vi "test6.4-RegisterInterruptAsStatusFromNonCSM.vi"(8 "error in (no error)":errorcluster, 11 "TestCase in":refnum<class "testcase-CSMBroadcast.lvclass">) -> (0 "error out":errorcluster, 3 "TestCase out":refnum<class "testcase-CSMBroadcast.lvclass">)   [LabVIEW 2017, in "testcase-CSMBroadcast.lvclass"]
uses:
  testcase-CSMBroadcast.lvclass
  src/user.lib/_NEVSTOP/Communicable State Machine(CSM)/AdvanceAPI/CSM - Broadcast Message Type.ctl
  <vilib>/addons/_JKI Toolkits/VI Tester/TestCase.llb/TestCase.lvclass
  src/user.lib/_NEVSTOP/Communicable State Machine(CSM)/Communicable State Machine.lvlib
  CSM/CSM-Testcase.lvlib
  C:/Program Files (x86)/National Instruments/LabVIEW 2017/vi.lib/addons/_JKI Toolkits/VI Tester/TestCase.llb/TestCase.lvclass
panel:
  out "output cluster":T1
  out "LoopCount":i32
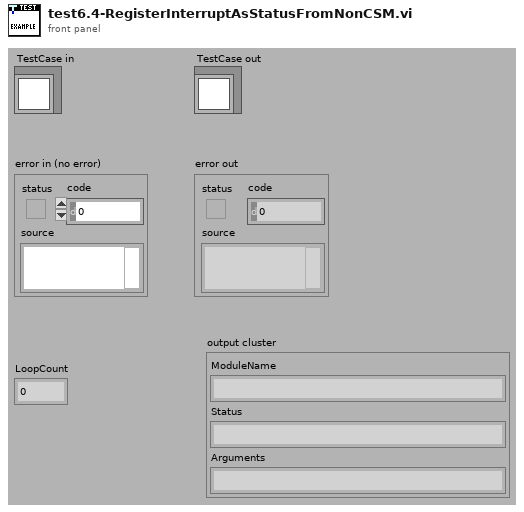
[diagram p1: front panel]
types:
  T1 = cluster{"ModuleName":string, "Status":string, "Arguments":string}
  T2 = typedef "Communicable State Machine.lvlib/CSM - Broadcast Message Type.ctl" = enum16{"<Null>", "Status", "Interrupt"}
  T3 = cluster{"Status Event":refnum<user-event>, "Interrupt Event":refnum<user-event>}
  T4 = cluster{"cluster":cluster{"ModuleName":string, "Status":string, "Arguments":string}}
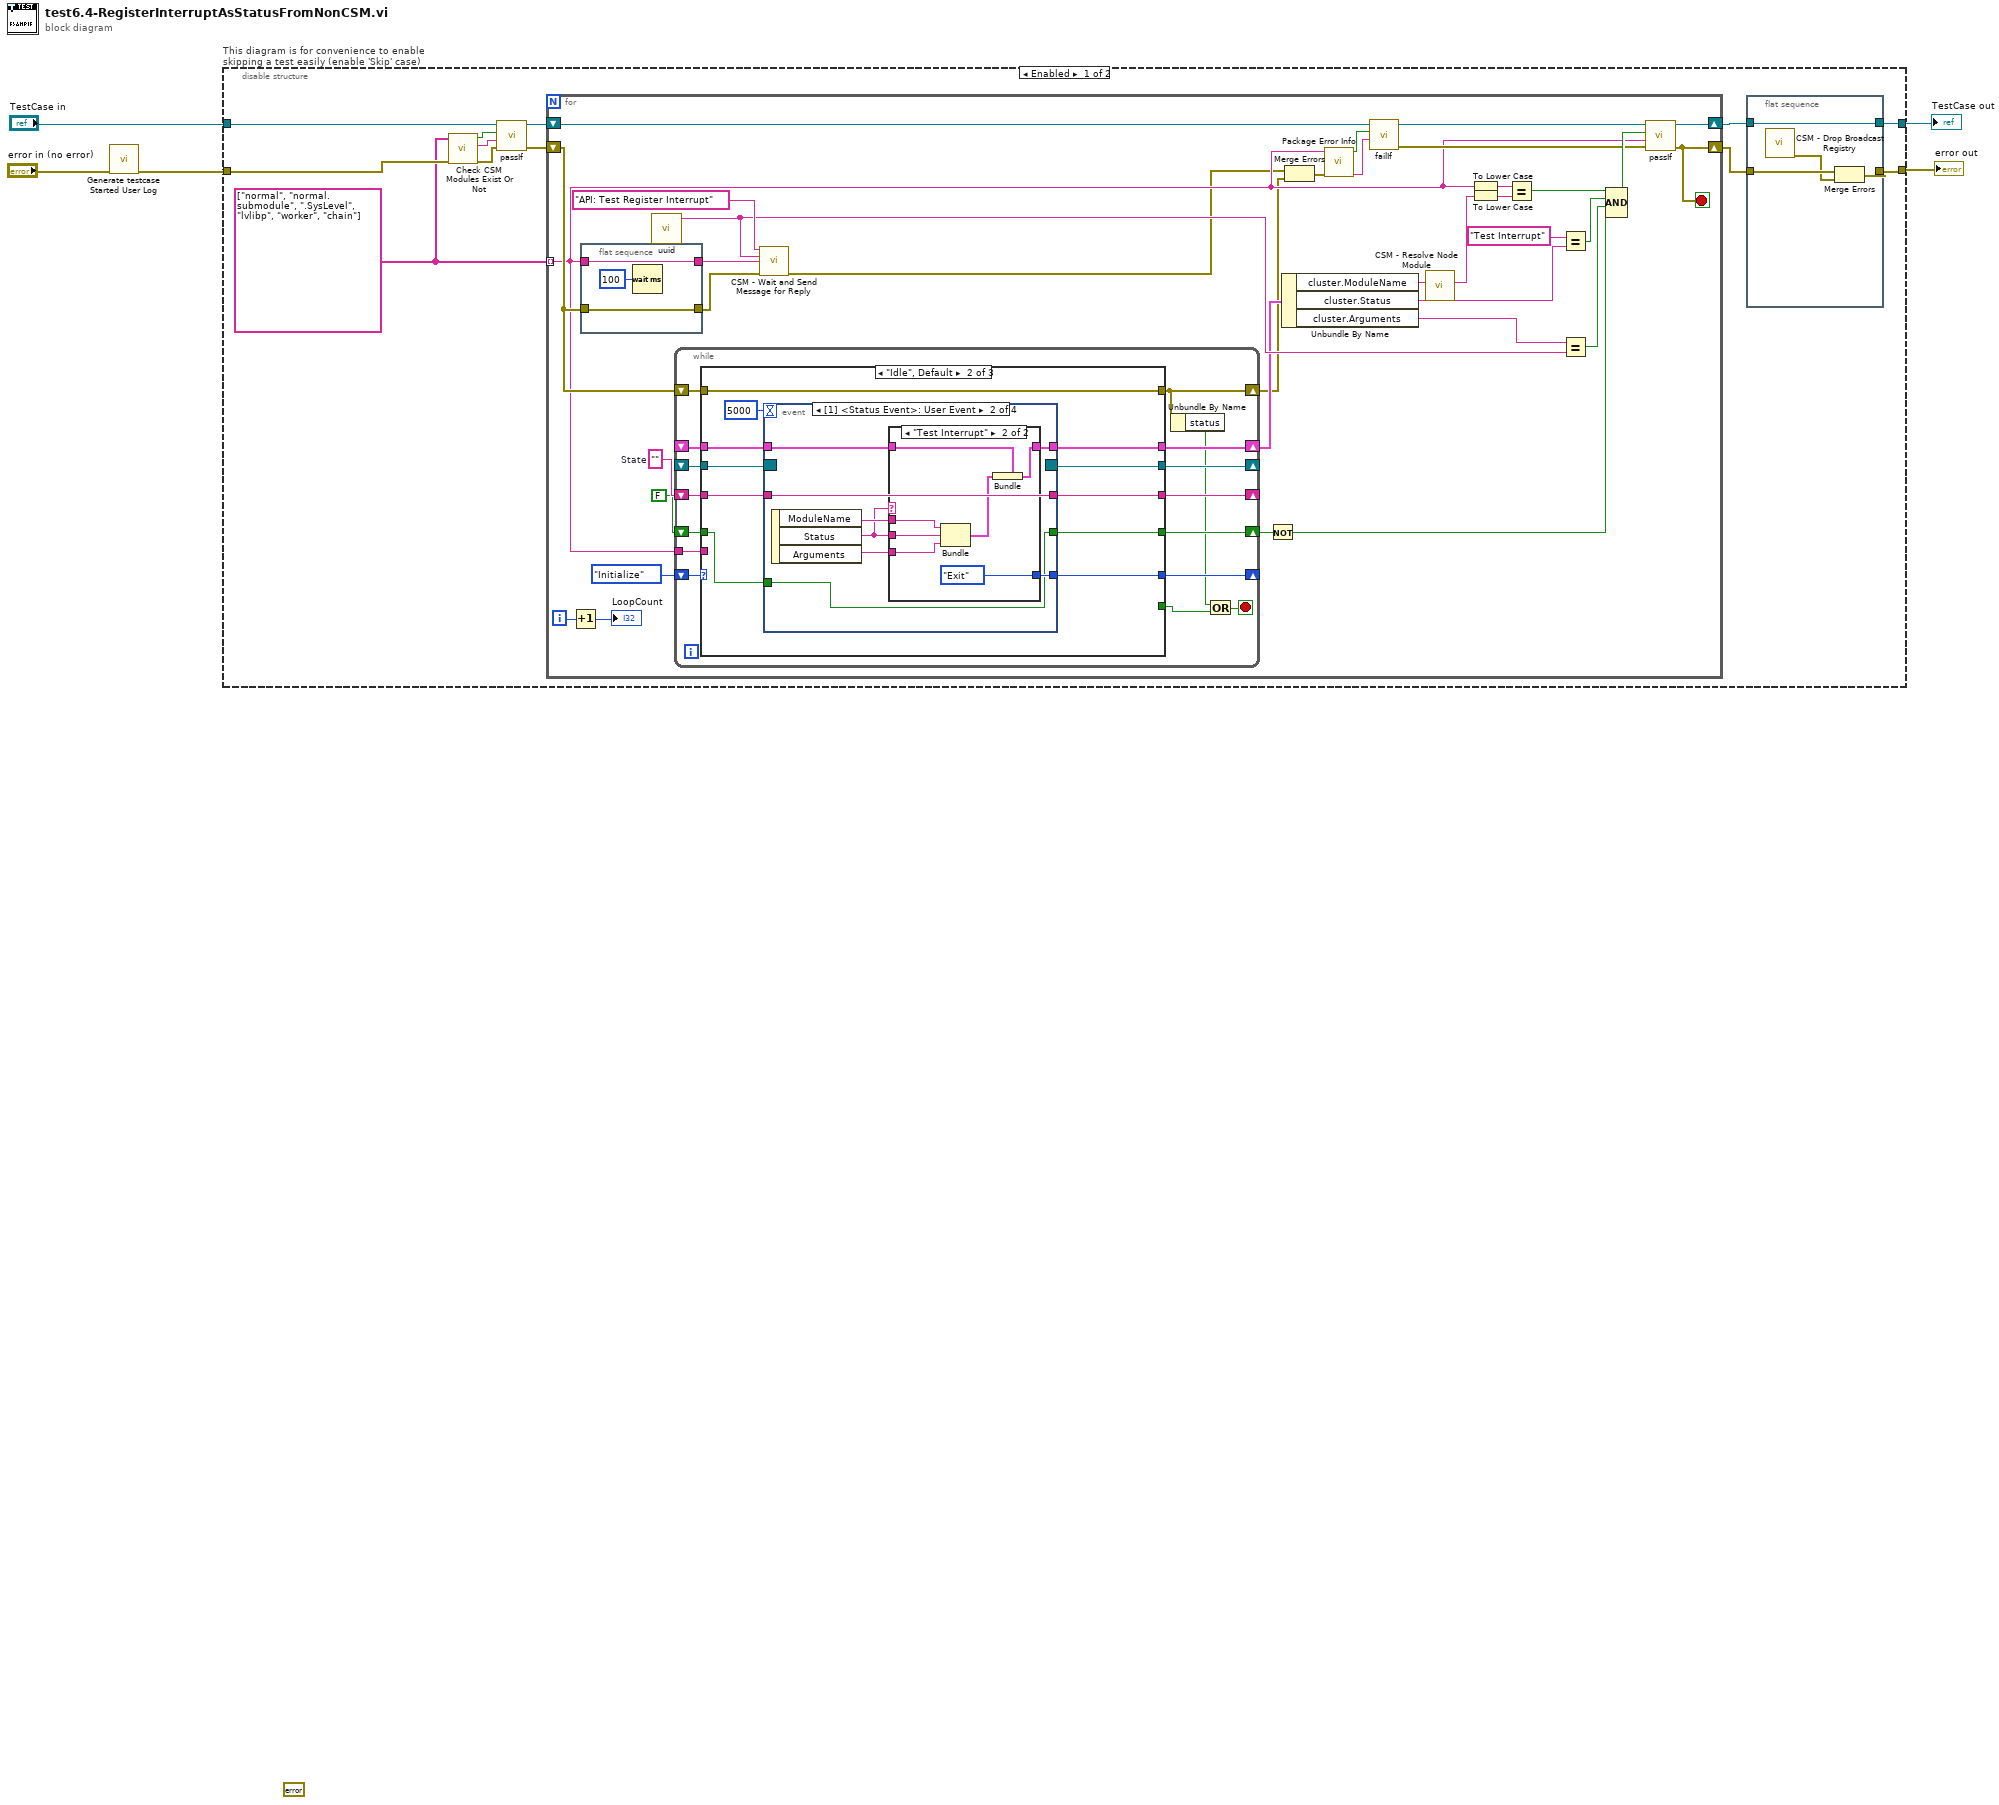
[diagram p0: block diagram]
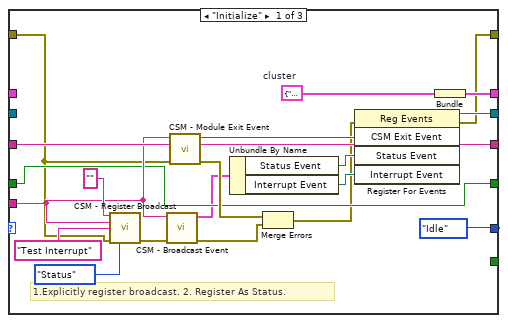
[diagram p2: hidden frame]
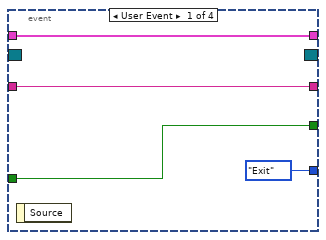
[diagram p3: hidden frame]
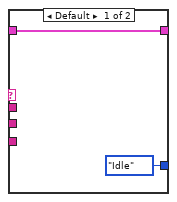
[diagram p4: hidden frame]
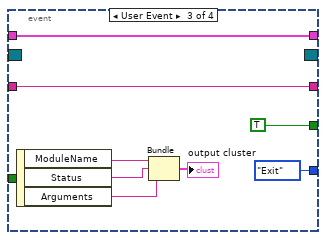
[diagram p5: hidden frame]
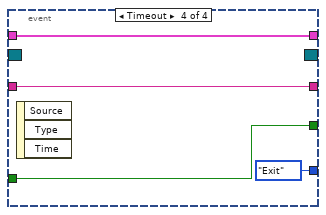
[diagram p6: hidden frame]
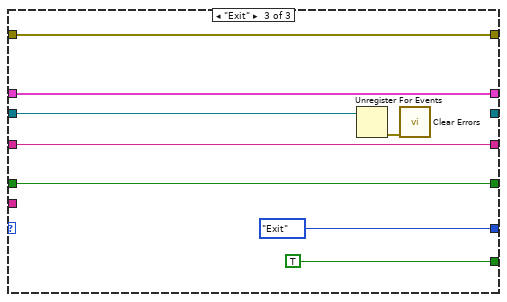
[diagram p7: hidden frame]
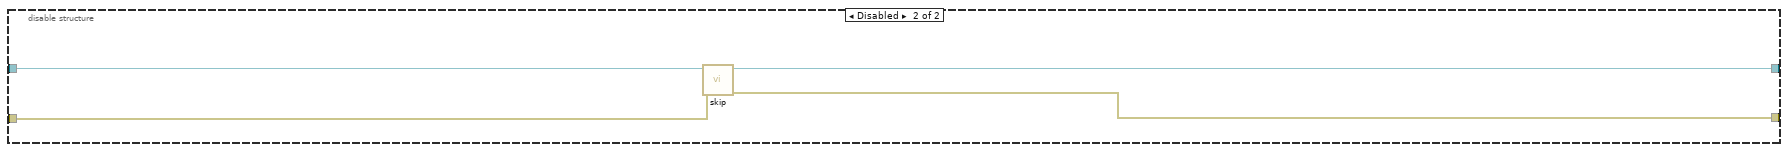
[diagram p8: hidden frame]
diagram:
  (unwired) errorcluster {"status"=FALSE, "code"=0, "source"=""} ("error out")
  n1 = call "Generate testcase Started User Log.vi"("Error In"="error in (no error)") -> ("error out"=w1:errorcluster)  [unwired: 10 in]
  n2 = disable-structure "This diagram is for convenience to enable skipping a test easily (enable 'Skip' case)" shown="Enabled" {
    disable-tunnel: "TestCase in" -> [w14 w151]
    disable-tunnel: [w7 w149] -> w3
    disable-tunnel: [w6 w150] -> w2
    disable-tunnel: w1 -> [w11 w148]
    frame Enabled {
      w10 = string[] ["normal", "normal.submodule", ".SysLevel", "lvlibp", "worker", "chain"]
      n3 = call "Check CSM Modules Exist Or Not.vi"("error in"=w11, "CSM names in"=w10) -> ("error out"=w15:errorcluster, "Debug string"=w16:string, "All Modules Exist?"=w17:bool)  [unwired: 7 in]
      n4 = call-dynamic "passIf.vi"("error in (no error)"=w15, "message (\"\")"=w16, "pass"=w17, "TestCase in"=w14) -> ("error out"=w12:errorcluster, "TestCase out"=w13:refnum<class "testcase-CSMBroadcast.lvclass">)  [unwired: 6 in]
      n5 = for {
        shift-right: [w48] -> w9
        shift-left: w13 -> [w28]
        tunnel: w10 -> [w24] mode=indexing
        shift-right: [w41] -> w8
        shift-left: w12 -> [w31]
        i -> [w43]
        stop <- w41 stop-if-true
        w55 = ""  # State
        n6 = Increment(x=w43) -> (x+1=→"LoopCount":i32)
        n7 = flat-sequence {
          tunnel: w24 -> [w59]
          tunnel: [w59] -> w53
          tunnel: w31 -> [w57]
          tunnel: [w57] -> w32
          frame #0 {
            n8 = Wait (ms)(milliseconds to wait=u32 100) -> ()  [unwired: 1 out]
          }
        }
        n9 = call "uuid.vi"() -> ("UUID"=w50:string)  [unwired: 11 in]
        n10 = while {
          shift-right: [w74] -> _
          shift-left: enum16{"Idle", "Initialize", "Exit"}."Initialize" -> [w75]
          shift-right: [w72] -> _
          shift-left: w55 -> [w73]
          shift-right: [w71] -> _
          shift-left: _ -> [w70]
          shift-right: [w69] -> w40
          shift-left: _ -> [w68]
          tunnel: w24 -> [w67]
          shift-right: [w66] -> w35
          shift-left: FALSE -> [w65]
          shift-right: [w63] -> w22
          shift-left: w31 -> [w64]
          stop <- w62 stop-if-true
          n11 = case shown="\"Idle\", Default" w75 {
            tunnel: [enum16{"Idle", "Initialize", "Exit"}."Idle" w106 enum16{"Idle", "Initialize", "Exit"}."Exit"] -> w74
            tunnel: [_ _ TRUE] -> w60
            tunnel: w73 -> [w94 w104 w145]
            tunnel: [w94 w105 w145] -> w72
            tunnel: [w92 w102 _] -> w71
            tunnel: w70 -> [_ w103 w144]
            tunnel: [w91 w100 w142] -> w69
            tunnel: w68 -> [_ w101 w142]
            tunnel: w67 -> [w84 _ _]
            tunnel: [w81 w98 w141] -> w66
            tunnel: w65 -> [w81 w97 w141]
            tunnel: w64 -> [w78 w96 w140]
            tunnel: [w76 w96 w140] -> w63
            frame "Initialize" {
              w90 = T1 {"ModuleName"="", "Status"="", "Arguments"=""}  # cluster
              # "1.Explicitly register broadcast. 2. Register As Status."
              n12 = call "CSM - Register Broadcast.vi"("CSM Name(Empty for Broadcast Event)"="", "Source CSM Name (* as Default)"=w84, "Trigger"="Test Interrupt" ("State"), "Error In"=w78, "Priority (No Change)"=CSM_-_Broadcast_Message_Type."Status" ("Priority(No Change)")) -> ("error out"=w86:errorcluster)  [unwired: 9 in, 1 out]
              n13 = call "CSM - Broadcast Event.vi"("Error In"=w86, "CSM Module"=w84) -> ("error out"=w88:errorcluster, "Broadcast Event"=w80:T3)  [unwired: 7 in, 1 out]
              n14 = call "CSM - Module Exit Event.vi"("Error In"=w78, "Name (\"\" to Use UUID) In"=w84) -> ("error out"=w89:errorcluster, "CSM Exit Event"=w93:refnum<user-event>)  [unwired: 7 in, 1 out]
              n15 = Unbundle By Name(w80) -> ("Status Event"=w83:refnum<user-event>, "Interrupt Event"=w82:refnum<user-event>)
              n16 = Merge Errors(w89, w88) -> (w77:errorcluster)
              n17 = register-events(error in=w77, w93, w83, w82) -> (reference out=w92:refnum<event-registration>, error out=w76:errorcluster)  [unwired: 1 in]
              n18 = Bundle("cluster"=w90) -> (w91:T4)  [unwired: 1 in]
            }
            frame "Idle", Default {
              n19 = event shown="[1] <Status Event>: User Event" {
                selector: w103 -> [_ _ _ _]
                dyn-events: [_ _ _ _] -> w102
                timeout: 5000 -> [_ _ _ _]
                tunnel: [enum16{"Idle", "Initialize", "Exit"}."Exit" w117 enum16{"Idle", "Initialize", "Exit"}."Exit" enum16{"Idle", "Initialize", "Exit"}."Exit"] -> w106
                tunnel: w104 -> [w110 w118 w135 w139]
                tunnel: [w110 w118 w135 w139] -> w105
                tunnel: w101 -> [w108 w114 w134 w138]
                tunnel: [w108 w113 w134 w138] -> w100
                tunnel: [w107 w111 TRUE w136] -> w98
                tunnel: w97 -> [w107 w111 _ w136]
                event User Event {
                  n20 = event-data() -> ()  [unwired: 1 in, 1 out]
                }
                event User Event {
                  n21 = event-data() -> ("ModuleName"=w116:string, "Status"=w112:string, "Arguments"=w115:string)  [unwired: 1 in]
                  n22 = case shown="\"Test Interrupt\"" w112 {
                    tunnel: [enum16{"Idle", "Initialize", "Exit"}."Idle" enum16{"Idle", "Initialize", "Exit"}."Exit"] -> w117
                    tunnel: w116 -> [_ w126]
                    tunnel: w112 -> [_ w125]
                    tunnel: w115 -> [_ w124]
                    tunnel: w114 -> [w120 w123]
                    tunnel: [w120 w121] -> w113
                    frame Default {
                    }
                    frame "Test Interrupt" {
                      n23 = Bundle("ModuleName"=w126, "Status"=w125, "Arguments"=w124) -> (w122:T1)  [unwired: 1 in]
                      n24 = Bundle(cluster=w123, "cluster"=w122) -> (w121:T4)
                    }
                  }
                }
                event User Event {
                  n25 = event-data() -> ("ModuleName"=w131:string, "Status"=w130:string, "Arguments"=w129:string)  [unwired: 1 in]
                  n26 = Bundle("ModuleName"=w131, "Status"=w130, "Arguments"=w129) -> (→"output cluster":T1)  [unwired: 1 in]
                }
                event Timeout {
                  n27 = event-data() -> ()  [unwired: 1 in, 3 out]
                }
              }
            }
            frame "Exit" {
              n28 = Unregister For Events(event registration refnum=w144) -> (error out=w143:errorcluster)  [unwired: 1 in]
              n29 = call <vilib>:"Clear Errors.vi"("error in (no error)"=w143) -> ()  [unwired: 5 in, 2 out]
            }
          }
          n30 = Unbundle By Name(w63) -> ("status"=w61:bool)
          n31 = Or(x=w61, y=w60) -> (x .or. y?=w62:bool)
        }
        n32 = call "CSM - Wait and Send Message for Reply.vi"("State"="API: Test Register Interrupt", "Arguments (\"\")"=w50, "Target Module"=w53, "Error In (No Error)"=w32) -> ("error out"=w23:errorcluster)  [unwired: 8 in, 3 out]
        n33 = Not(x=w35) -> (.not. x?=w34:bool)
        n34 = Unbundle By Name(w40) -> ("cluster.ModuleName"=w38:string, "cluster.Status"=w51:string, "cluster.Arguments"=w49:string)
        n35 = Merge Errors(w23, w22) -> (w29:errorcluster)
        n36 = call "Package Error Info.vi"("error in"=w29, "String in"=w24) -> ("packed error info out"=w30:string, "error status"=w25:bool)  [unwired: 8 in]
        n37 = call-dynamic "failIf.vi"("message (\"\")"=w30, "fail"=w25, "TestCase in"=w28) -> ("error out"=w26:errorcluster, "TestCase out"=w27:refnum<class "testcase-CSMBroadcast.lvclass">)  [unwired: 7 in]
        n38 = call "CSM - Resolve Node Module.vi"("Node Name"=w38) -> ("CSM Module Name"=w36:string)  [unwired: 10 in]
        n39 = To Lower Case(string=w24) -> (all lower case string=w39:string)
        n40 = To Lower Case(string=w36) -> (all lower case string=w37:string)
        n41 = Equal?(x=w39, y=w37) -> (x = y?=w47:bool)
        n42 = Equal?(x="Test Interrupt" ("State"), y=w51) -> (x = y?=w46:bool)
        n43 = Equal?(x=w49, y=w50) -> (x = y?=w45:bool)
        n44 = Compound Arithmetic op=AND(w47, w46, w45, w34) -> (w44:bool)
        n45 = call-dynamic "passIf.vi"("error in (no error)"=w26, "message (\"\")"=w24, "pass"=w44, "TestCase in"=w27) -> ("error out"=w41:errorcluster, "TestCase out"=w48:refnum<class "testcase-CSMBroadcast.lvclass">)  [unwired: 6 in]
      }
      n46 = flat-sequence {
        tunnel: w8 -> [w21]
        tunnel: [w20] -> w6
        tunnel: w9 -> [w18]
        tunnel: [w18] -> w7
        frame #0 {
          n47 = call "CSM - Drop Broadcast Registry.vi"() -> ("error out"=w19:errorcluster)  [unwired: 15 in]
          n48 = Merge Errors(w21, w19) -> (w20:errorcluster)
        }
      }
    }
    frame Disabled {
      # "skip test result while test is under development"
      n49 = call <vilib>:"skip.vi"("error in (no error)"=w148, "TestCase in"=w151) -> ("error out"=w150:errorcluster, "TestCase out"=w149:refnum<class "testcase-CSMBroadcast.lvclass">)  [unwired: 8 in]
    }
  }
  "error out" <- w2
  "TestCase out" <- w3
